vi "Read Value (variant).vi"(8 "error in (no error)":errorcluster, 11 "String D Element in":refnum<class "String D Element.lvclass">) -> (0 "error out":errorcluster, 2 "Variant":variant, 3 "String D Element out":refnum<class "String D Element.lvclass">)   [LabVIEW 2018, in "D Datagrid Library.lvlib" / "String D Element.lvclass"]
uses:
  String D Element.lvclass
  String D Element.lvclass/String D Element.ctl
  Read Value.vi
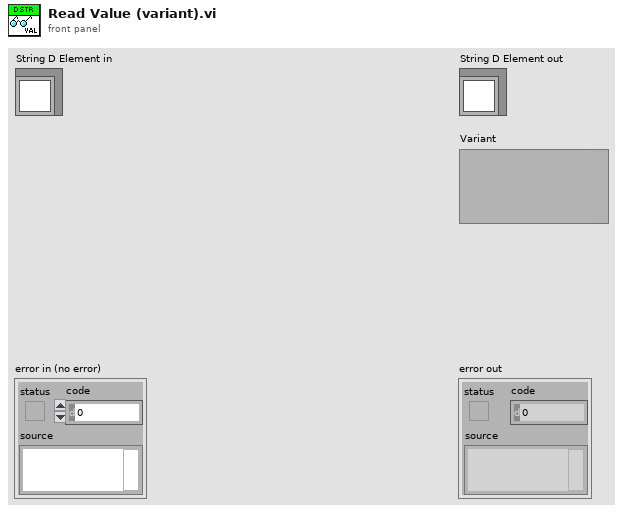
[diagram p1: front panel]
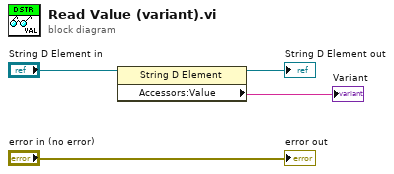
[diagram p0: block diagram]
diagram:
  n1 = property class="String D Element"(reference="String D Element in") -> (reference out=→"String D Element out":refnum<class "String D Element.lvclass">, "Accessors:Value"=→"Variant":string)  [unwired: 1 in, 1 out]
  "error out" <- "error in (no error)"
